vi "Load MC vis setting.vi"(8 "error in":errorcluster) -> (0 "error out":errorcluster, 3 "MC Visible?":bool)   [LabVIEW 2017]
uses:
  Typedefs/Which path.ctl
  <vilib>/Utility/config.llb/NI_LVConfig.lvlib
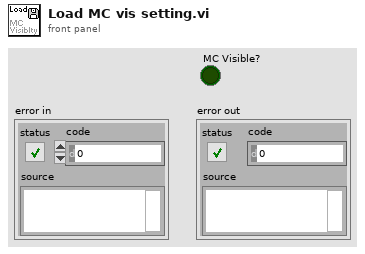
[diagram p1: front panel]
types:
  T1 = typedef "Which path.ctl" = enum16{"Configuration Files", "Calibration Files", "Images", "Setup.ini", "Loaded User profile.ini", "User's-Previous session.ini", "New user profile.ini", "Selected User profile.ini", "User profiles folder", "Power meter scaling.txt", "FOV Cal.ini", "Calibration.ini"}
  T2 = typedef "NI_LVConfig.lvlib/Config Data RefNum.ctl" = refnum<k1>
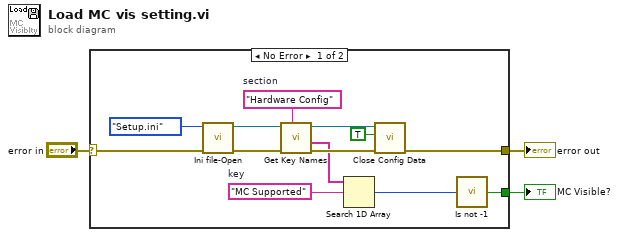
[diagram p0: block diagram]
diagram:
  n1 = case shown="No Error" "error in" {
    selector: "error in" -> [w12 w17]
    tunnel: [w15 w17] -> w3
    tunnel: [w6 _] -> w1
    frame No Error {
      w5 = "Hardware Config"  # section
      w8 = "MC Supported"  # key
      n2 = call "Ini file-Open.vi"("Error In"=w12, "Which file?"=Which_path."Setup.ini") -> ("error out"=w11:errorcluster, "User profile ini file ref"=w14:T2)  [unwired: 6 in, 2 out]
      n3 = call <vilib>:"Get Key Names.vi"("section"=w5, "error in (no error)"=w11, "refnum"=w14) -> ("error out"=w13:errorcluster, "key names"=w9:string[], "refnum out"=w10:T2)  [unwired: 5 in, 1 out]
      n4 = Search 1D Array(1D array=w9, element=w8) -> (index of element=w7:i32)  [unwired: 1 in]
      n5 = call <vilib>:"Close Config Data.vi"("error in (no error)"=w13, "write file if changed (T)"=TRUE ("write configuration file? (F)"), "refnum"=w10) -> ("error out"=w15:errorcluster)  [unwired: 7 in, 1 out]
      n6 = call <userlib>:"Is not -1.vi"("x"=w7) -> ("x != -1?"=w6:bool)  [unwired: 4 in]
    }
    frame Error {
    }
  }
  "error out" <- w3
  "MC Visible?" <- w1
